vi "RFLoopback.vi"(6 "xsrpip":string, 7 "pcip":string, 8 "error in":errorcluster, 10 "txdataIQ":cdb[](array[numeric]), 11 "Path In":path) -> (0 "error out":errorcluster, 1 "ERR_CODE":dbl format="%#_13g", 2 "rxdataIQ":cdb[](array[numeric]), 3 "Path Out":path)   [LabVIEW 2015]
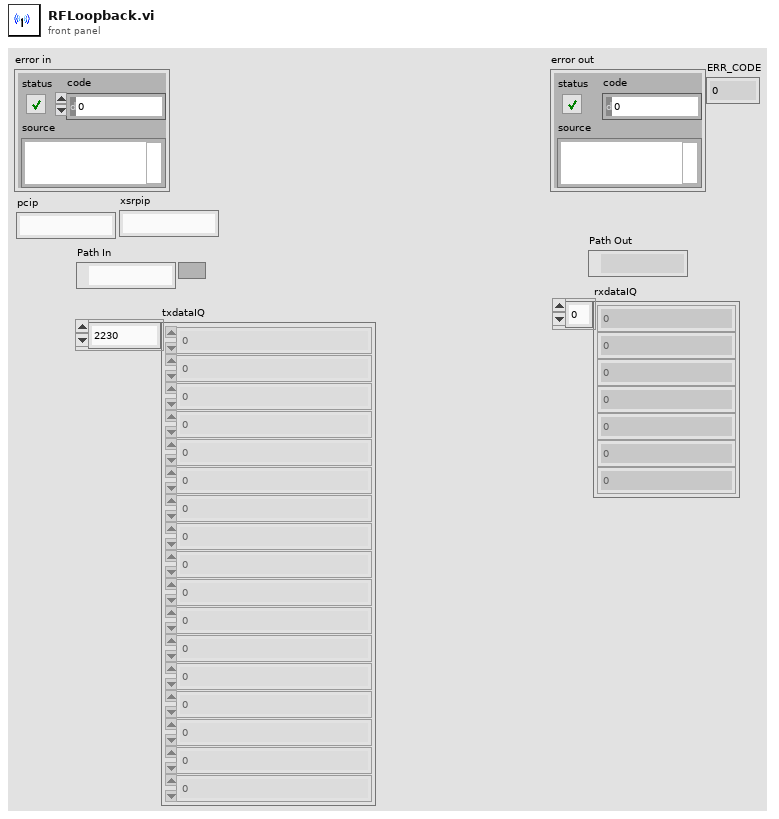
[diagram p1: front panel]
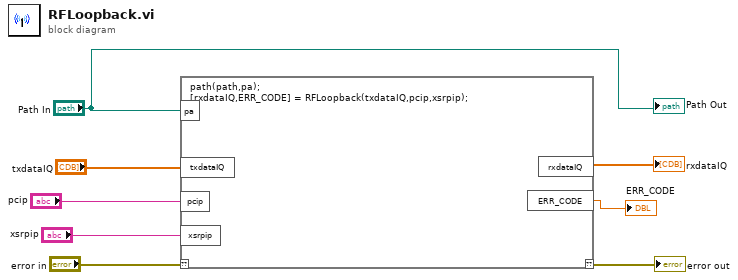
[diagram p0: block diagram]
diagram:
  n1 = script code="path(path,pa);\n[rxdataIQ,ERR_CODE] = RFLoopback(txdataIQ,pcip,xsrpip);"("??"="error in", "pa"="Path In", "txdataIQ"="txdataIQ", "pcip"="pcip", "xsrpip"="xsrpip") -> ("??"=→"error out":errorcluster, "rxdataIQ"=→"rxdataIQ":cdb[], "ERR_CODE"=→"ERR_CODE":dbl)
  "Path Out" <- "Path In"
